vi "Set Visible State on Multiple Controls.vi"(8 "error in":errorcluster, 10 "Hide?":bool[](array[boolean]), 11 "Control Refnums":refnum<vi>[](array[refnum])) -> (0 "error out":errorcluster, 3 "Dup Control Refnums":refnum<vi>[](array[refnum]))   [LabVIEW 2022 SP3, in "EDT VIE.lvlib"]
uses:
  EDT VIE.lvlib
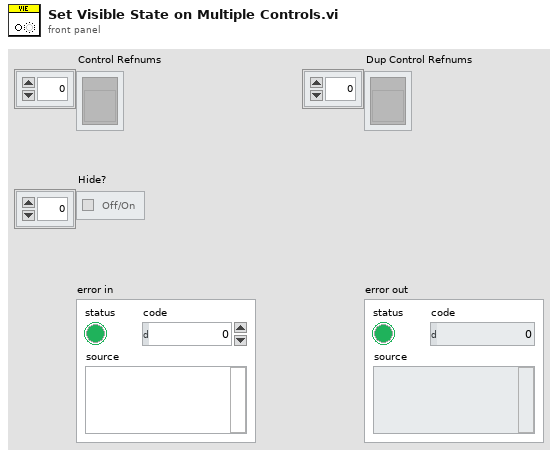
[diagram p1: front panel]
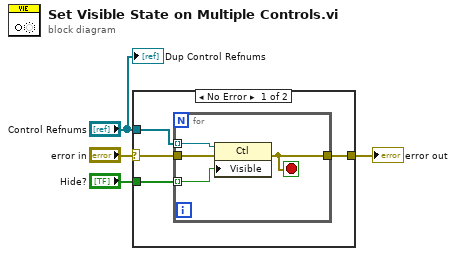
[diagram p0: block diagram]
diagram:
  n1 = case shown="No Error" "error in" {
    selector: "error in" -> [w7 w13]
    tunnel: "Control Refnums" -> [w8 _]
    tunnel: [w6 w13] -> w3
    tunnel: "Hide?" -> [w5 _]
    frame No Error {
      n2 = for {
        tunnel: w8 -> [w12] mode=indexing
        tunnel: w7 -> [w11]
        tunnel: [w9] -> w6
        tunnel: w5 -> [w10] mode=indexing
        stop <- w9 stop-if-true
        n3 = property class="Ctl"(reference=w12, error in=w11, "Visible"=w10) -> (error out=w9:errorcluster)  [unwired: 1 out]
      }
    }
    frame Error {
    }
  }
  "error out" <- w3
  "Dup Control Refnums" <- "Control Refnums"
